vi "Ch Get Type.vi"(9 "Type":string, 10 "Channel":u8, 11 "devId":i32) -> (1 "Type out":string, 2 "devId out":i32, 3 "function return":i32)   [LabVIEW 2013, in "CHR34XXX.lvlib"]
doc: "DLL BOOL __stdcall CHR34XXX_Ch_SetType(IN int devId,IN BYTE Channel,IN BYTE Type); DLL BOOL __stdcall CHR34XXX_Ch_GetType(IN int devId,IN BYTE Channel,OUT BYTE *Type);"
uses:
  CHR34XXX.lvlib
  CHR34XXX.dll
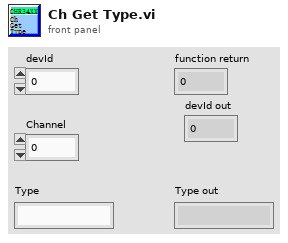
[diagram p1: front panel]
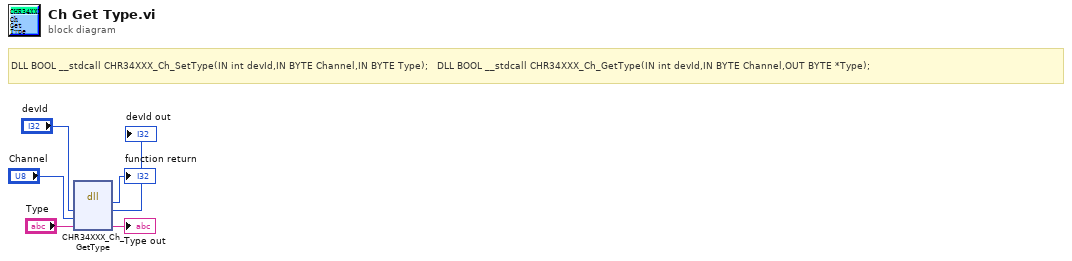
[diagram p0: block diagram]
diagram:
  # "DLL BOOL __stdcall CHR34XXX_Ch_SetType(IN int devId,IN BYTE Channel,IN BYTE Type);   DLL BOOL __stdcall CHR34XXX_Ch_GetType(IN int devId,IN BYTE Channel,OUT BYTE *Type);"
  n1 = dll-call lib="C:/Users/Administrator/Desktop/CHR34XXX_lv/lv_lib/CHR34XXX.*" fn="CHR34XXX_Ch_GetType"("devId"="devId", "Channel"="Channel", "Type"="Type") -> (→"function return":i32, "devId"=→"devId out":i32, "Type"=→"Type out":string)  [unwired: 4 in, 2 out]
